vi "AlliGator Decay Fit Parameter Map Actions.vi"(0 "AlliGator Q Elements in":T4[](array[typedef]), 1 "VI in":refnum<vi>, 2 "Script in":bool, 5 "data value reference":refnum<data-value>, 7 "AlliGator Q Event in":T5=enum."GUI:Idle", 9 "Data":variant, 11 "error in (no error)":errorcluster, 12 "AlliGator Ctrl Refnums":T6) -> (3 "Script out":bool, 4 "AlliGator Q Elements out":T4[](array[typedef]), 6 "Data Value Reference out":refnum<data-value>, 10 "[Notebook Message]":T1[](array[typedef]) {"Message Style"."Text Alignment" items=["Left", "Right", "Center"]}, 15 "error out":errorcluster)   [LabVIEW 2021, in "AlliGator Action Engine.lvlib"]
doc: "Processes AlliGator decay fit parameter map-related actions."
uses:
  AlliGator Action Engine.lvlib
  AlliGator Internal Variables v2.ctl
  <vilib>/vision/Image Controls.llb/IMAQ Image.ctl
  AlliGator Gate Image Set.ctl
  AlliGator FLI Dataset Type.ctl
  AlliGator Data Series Type.ctl
  AlliGator Dataset Channel.ctl
  AlliGator Gate Arithmetic.ctl
  AlliGator Displayed Image.ctl
  Image/Named ROI Description.ctl
  AlliGator Decay Metadata v3.ctl
  AlliGator Decay Background Subtraction Info.ctl
  AlliGator Baseline Subtraction Method.ctl
  Graphs/XY Graph/XY Graph Plot Shift Parameters.ctl
  Graphs/XY Graph/XY Graph Plot Shift Method.ctl
  AlliGator Decay Extrapolation Parameters.ctl
  Phasor/Calibration Phasor (m, phi).ctl
  Phasor/Phasor Reference Series.ctl
  Phasor/Phasor Calibration Map v2.ctl
  Phasor/Phasor (g, s).ctl
  AlliGator Raw Phasor Plot Data v4.ctl
  Phasor/Phasor Standard Deviation Options.ctl
  AlliGator Phasor Multi-Harmonic Data.ctl
  Phasor/Phasor Harmonic Data.ctl
  AlliGator Decay Fit Options & Parameters v2.ctl
  Fits/IRF(X)PSED/Decay Fit Options v2.ctl
  Fits/Decay Convolution/Decay Model.ctl
  Fits/Residual Type.ctl
  Fits/IRF(X)PSED/Fit Weights Type.ctl
  Fits/Non-linear Fitting Method v2.ctl
  Fits/Fit Calculation Method.ctl
  Fits/Non-linear Fitting Algorithm.ctl
  AlliGator Decay Fit Parameter Constraints 2.ctl
  Fits/IRF(X)PSED/Decay Fit Parameters In List.ctl
  Fits/IRF(X)PSED/MLE Baseline Offset Type.ctl
  AlliGator Decay Preprocessing Parameters.ctl
  Fits/IRF(X)PSED/Decay Fit Parameters & Derived Quantities List.ctl
  AlliGator Q Event.ctl
  AlliGator Ctrl Refnums.ctl
  AlliGator Other Ctrl Refnums.ctl
  AlliGator State Indicator.ctl
  AlliGator Phasor Plot Ctrl Refnums.ctl
  AlliGator Phasor Graph Ctrl Refnums.ctl
  Phasor/Phasor Calibration Type.ctl
  AlliGator Dataset Ctrl Refnums.ctl
  AlliGator Registered Events Ctrl Refnums.ctl
  AlliGator Image Histogram Control Refnums.ctl
  Histograms/Linear Histogram Options.ctl
  Histograms/Histogram Bin Option.ctl
  Histograms/Histogram Bin Position.ctl
  AlliGator Decay Fit Map Control Refnums.ctl
  AlliGator Q Element.ctl
  Notebook/Notebook Message Object.ctl
  Rich Text Box/Text Formatting.ctl
  Rich Text Box/Text Colors.ctl
  Alligator Elements Order in Action Stack.ctl
  AlliGator Variables List.ctl
  AlliGator Image Display Type.ctl
  Palette/Image Palette Information.ctl
  Image/Image Display Palette Type.ctl
  Files/Load-Save File Info.ctl
  c5217346-0728-4db9-a30e-52dae72b7cfc.vi
  Variant/Variant to Data/Variant to Boolean.vi
  AlliGator Add Single Action to Stack.vi
  Variant/Variant to Data/Variant to [String].vi
  Variant/Variant to Data/Variant to String.vi
  Variant/Variant to Data/Variant to I32.vi
  AlliGator Local Decay Window.lvlib
  Fits/Fits.lvlib
  Rich Text Box/Rich Text Box.lvlib
  GUI/GUI.lvlib
  AlliGator Decay Fit Parameter Map.lvlib
  Variant/Variant to Data/Variant to Data.lvlib
  AlliGator Globals, Variables & Constants.lvlib
  Palette/Palette.lvlib
  AlliGator GUI.lvlib
  Image/Image.lvlib
  AlliGator Files.lvlib
  AlliGator Internal Variables.lvlib
  Files/Files.lvlib
  Sound/Sound.lvlib
  Phasor/Phasor.lvlib
  AlliGator Decay Preprocessing.lvlib
  Graphs/XY Graph/XY Graph Add-Ons.lvlib
  AlliGator Phasor Graph.lvlib
  AlliGator Phasor Plot.lvlib
  AlliGator Source Image.lvlib
  AlliGator Decay Fit.lvlib
  AlliGator Settings.lvlib
  AlliGator Dual-Channel Datasets.lvlib
  Histograms/Histogram Window.lvlib
  Notebook/Notebook.lvlib
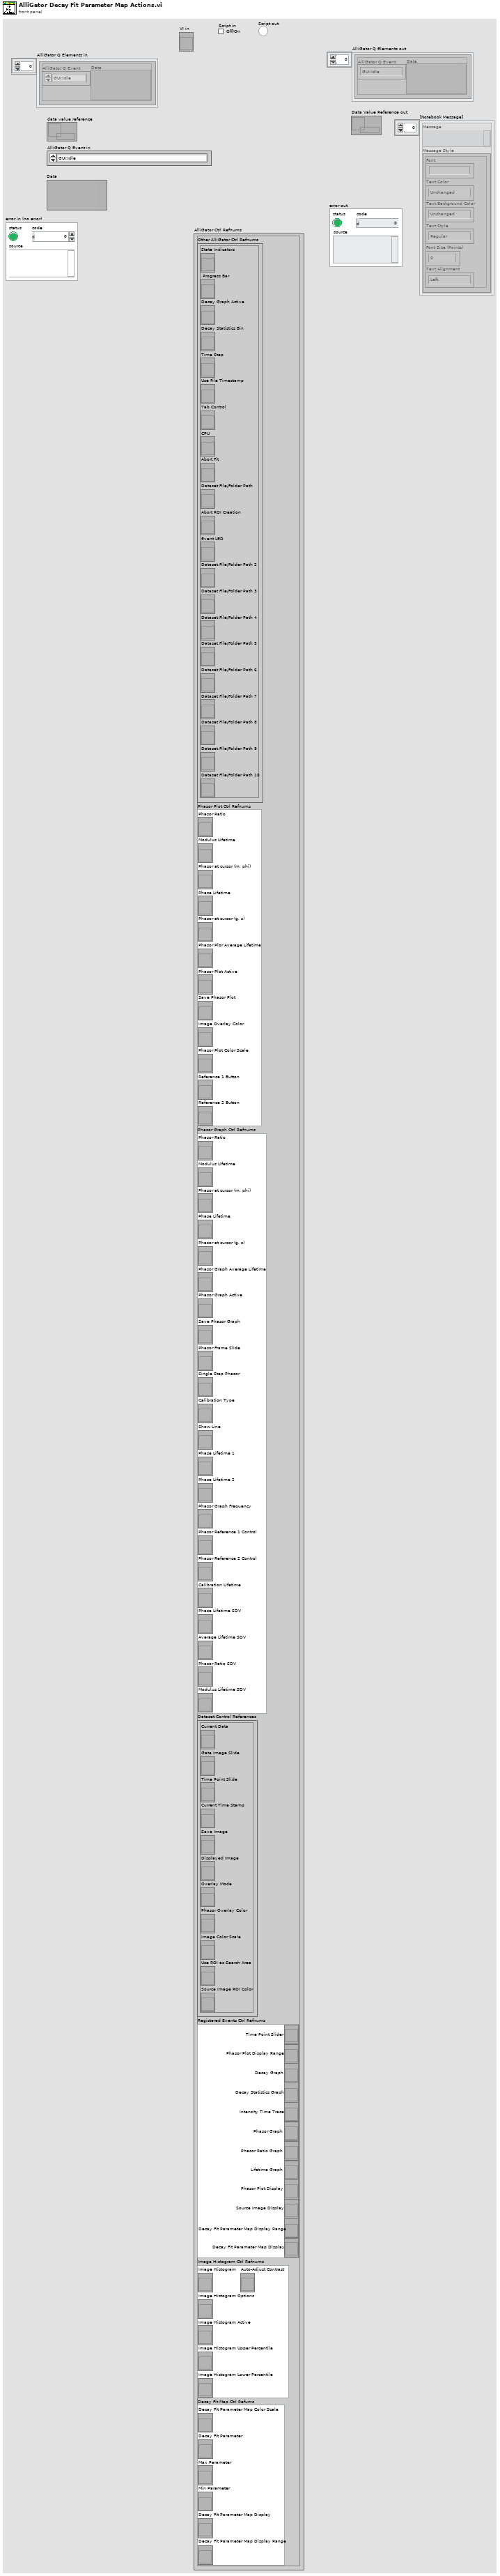
[diagram p1: front panel]
types:
  T1 = typedef "Notebook.lvlib/Notebook Message Object.ctl" = cluster{"Message":string, "Message Style":T2}
  T2 = typedef "Rich Text Box.lvlib/Text Formatting.ctl" = cluster{"Font":string, "Text Color":T3, "Text Background Color":T3, "Text Style":enum16{"Regular", "Bold", "Italic", "Underline", "Strikeout"}, "Font Size (Points)":dbl, "Text Alignment":i32}
  T3 = typedef "Rich Text Box.lvlib/Text Colors.ctl" = enum16{"Unchanged", "Black", "Blue", "Brown", "Gray", "Green", "Orange", "Pink", "Red", "White"}
  T4 = typedef "AlliGator Action Engine.lvlib/AlliGator Q Element.ctl" = cluster{"AlliGator Q Event":T5, "Data":variant}
  T5 = typedef "AlliGator Action Engine.lvlib/AlliGator Q Event.ctl" = enum16{"---- Files ----", "Files:Set Batch Export Files To Save", "Files:Set Dataset Loading & Pre-processing Options", "Files:Check #Frames in Dataset", "Files:Increment Frame Index", "Files:Open Mask Image", "Files:Open White Light Image", "Files:Open Single Dataset", "Files:New Folder of Folders Selected", "Files:Load File (all Types)_Scriptable", "Files:Move Flattened Series to Folders Series", "Files:Select Folder", "Files:Load FLI Dataset", "Files:Load Swiss SPAD 1 Dataset", "Files:Load Swiss SPAD 2 Dataset", "Files:Load .sdt FLI Dataset", "Files:Load .ptu FLI Dataset", "Files:Load .bin FLI Dataset", "Files:Load Single Gate Image Folder", "Files:Load I/m/phi Dataset (deprecated)", "Files:Load Single Image", "Files:Subtract Background File", "Files:Export FLI Dataset", "Files:Load HDF5 FLI Dataset", "Files:Set Destination File Path", "Files:Save Mask Image", "Files:Batch Conversion", "Files:New Folder Selected", "Files:Close FLI Dataset", "Files:Close FLI Dataset Series", "Files:Close White Light Image", "Files:Close Mask Image", "---- FLI Dataset ----", "FLI Dataset:Channel Arithmetic", "FLI Dataset:Export Average Lifetime Map as ASCII", "FLI Dataset:Export User-Defined Quantity Map as ASCII", "FLI Dataset:Python Function FLI Dataset Event", "FLI Dataset:ROI Analysis", "FLI Dataset:Tilted Logistic Square Gated IRF Characteristics Map", "FLI Dataset:Logistic Square Gated IRF Characteristics Map", "FLI Dataset:Square Gated IRF Characteristics Map", "FLI Dataset:Multi-ROI Single-Pixel Phasor Analysis", "FLI Dataset:Multi-ROI Single-Pixel NLSF Analysis", "FLI Dataset:All ROIs IRF Extraction", "FLI Dataset:All ROIs Decay Fit Non-Interactive (Fast + Individual IRF)", "FLI Dataset:All ROIs Phasor Analysis", "FLI Dataset:All ROIs Decay Fit", "FLI Dataset:Fluorescence Decay Statistics", "FLI Dataset:Update Decay Statistics Graph", "FLI Dataset:Get Decay from ROI", "FLI Dataset:All ROIs Average Lifetimes", "---- FLI Dataset Series ----", "FLI Dataset Series:Sum All Datasets in Series", "FLI Dataset Series:Add Dataset to Accumulated Dataset", "FLI Dataset Series:Display Accumulated Dataset", "FLI Dataset Series:Clear Dataset Series Sum", "FLI Dataset Series:Time-Series Analysis (NLSF)", "FLI Dataset Series:Time-Series Analysis (Phasor)", "---- Image ----", "Image:Update Image Profile Plots", "Image:Image Histogram Cursor Move", "Image:Image Histogram", "Image:Image Contrast", "Image:Set Image Histogram Cursor Move Flag", "Image:Clear Image Overlay", "Image:Use ROI as Search Area", "Image:Set ROI Diameter", "Image:Save Image Data as TIFF", "Image:Save Displayed Image with Overlay", "Image:Save Image Overlay Only", "Image:Save Image as Hot Pixel Mask", "Image:Change Source Image Color Palette", "Image:Copy Image to Clipboard", "Image:Source Image ROI Selection", "Image:Delete All ROIs", "Image:Delete All Unselected ROIs", "Image:Delete ROI", "Image:Merge All ROIs", "Image:Store ROI", "Image:Source Image ROI Storage", "Image:Export ROI Description to Notebook", "Image:Save ROI", "Image:Load ROI", "Image:Paste ROI Definition", "Image:Clear ROI", "Image:Identify ROIs in Mask Image", "Image:Create Complementary ROI", "Image:Create Contour ROI", "Image:Create ROI(s) from Pixels with Peak above Min_Scriptable", "Image:Create ROI(s) from Pixels with Intensity above Min_Scriptable", "Image:Compute ROI Statistics", "Image:Delete ROI(s) based on ROI Characteristics", "Image:Create ROI Grid", "Image:ROI to Individual Pixel ROIs", "Image:Python Function Source Image Event", "Image:Show Phasor Calibration Map ROI Centers", "Image:Convert ROI to Mask Image", "Image:Mouse Move", "Image:Mouse Up", "Image:Set Source Image Mouse Move Flag", "Image:Add Scale Bar Overlay", "Image:Delete Existing ROIs Option", "---- Decay ----", "Decay:Clear IRF/Reference Plot", "Decay:Clear Local IRFs", "Decay:Add Decay to Graph", "Decay:Smoothen Plot", "Decay:Smoothen Plot Tail", "Decay:Average Selected Plots", "Decay:Extract IRF", "Decay:Optimal IRF Extraction", "Decay:Threshold IRF", "Decay:Fit to Model IRF", "Decay:Fit IRF to Square Gate", "Decay:Fit IRF to Logistic Square Gate", "Decay:Fit IRF to Tilted Logistic Square Gate", "Decay:Create Bounding Cursors Set", "Decay:Export Bounding Cursors Definition to Notebook", "Decay:Denoise Plot", "Decay:Compute Cumulative Function", "Decay:Use as Reference Decay", "Decay:Show Reference Decay/IRF", "Decay:Extrapolate Decay", "Decay:Create Head & Tail Bounding Cursors", "Decay:Store Cursor-defined Head & Tail Fractions", "Decay:Rebin Plot", "Decay:1-Normalize Decay", "Decay:[0-1]-Normalize Plot", "Decay:Straighten Decay", "Decay:Shift Decay", "Decay:Fold Decay", "Decay:Fit Decay", "Decay:Global Fit of Selected Decays", "Decay:Post Global Fit Script", "Decay:Add Global Fit Parameters to Graph", "Decay:Add Decay Parameter(s) to Plot (Graph)", "Decay:Export Decay to Phasor Graph", "Decay:Plot Decay Shifts", "Decay:Compute Average Lifetime", "Decay:Plot Convolution", "Decay:Graph Tip Strip Update", "---- Decay Statistics ----", "Decay Statistics:Tip Strip Update", "---- Intensity Time Trace ----", "Intensity Time Trace:Use File Timestamp", "Intensity Time Trace:Load Intensity Corrections File", "Intensity Time Trace:Clear Intensity Corrections File", "Intensity Time Trace:Tip Strip Update", "---- Phasor Plot ----", "Phasor Plot:Build Phasor Plot", "Phasor Plot:Change Phasor Plot Color Palette", "Phasor Plot:Adjust Phasor Plot Display Range", "Phasor Plot:Highlight Image ROI in Phasor Plot", "Phasor Plot:Save Phasor Plot Image with Overlay", "Phasor Plot:Export Complex Phasor Map", "Phasor Plot:Export Phasor Ratio Map", "Phasor Plot:Export Average Lifetime Map", "Phasor Plot:Compute Phase Lifetime Histogram", "Phasor Plot:Compute Phasor Ratio Histogram", "Phasor Plot:Compute Phase Lifetime vs Intensity Scatter Plot", "Phasor Plot:Weber 2-Component Decomposition", "Phasor Plot:Update Phasor Color Map Vertices", "Phasor Plot:Clear Phasor Overlay", "Phasor Plot:Use Segment Extremities as References", "Phasor Plot:Use UC/Segment Intersections as References", "Phasor Plot:Use UC/Principal Axis Intersections as References", "Phasor Plot:Use UC/Linear Fit Intersections as References", "Phasor Plot:Update Phasor Plot Reference", "Phasor Plot:Show Local Phasor Info in Phasor Plot", "Phasor Plot:Update Phasor Plot State", "Phasor Plot:Phasor Plot ROI Storage", "Phasor Plot:Phasor Plot ROI Selection", "Phasor Plot:Python Function Phasor Plot Event", "Phasor Plot:Overlay Phasor ROI, Ratio or Map in Source Image", "Phasor Plot:Compute Decay of Selected Phasors", "Phasor Plot:Phasor at Image Pixel", "Phasor Plot:Mouse Move", "Phasor Plot:Mouse Up", "Phasor Plot:Display Range Mouse Move", "Phasor Plot:Set Mouse Move Flag", "---- Phasor Graph ----", "Phasor Graph:Calibrated Phasor Map Series", "Phasor Graph:Whole Image Phasor Scatter Plot (Todo)", "Phasor Graph:Get Phasor Value", "Phasor Graph:Create New Phasor Plot Dialog", "Phasor Graph:Update Last Phasor Value", "Phasor Graph:Update Phasor (m, phi)", "Phasor Graph:Remove Single Phasor from Plot", "Phasor Graph:Add Single Phasor to Plot", "Phasor Graph:Remove Phasor Plot", "Phasor Graph:Remove Selected Phasor Plots", "Phasor Graph:Clear Phasor Data", "Phasor Graph:Clear Phasor Graph", "Phasor Graph:Cursor Move", "Phasor Graph:Draw Cursor Connecting Line", "Phasor Graph:Clear Cursor Connecting Line", "Phasor Graph:Find UC Intersection", "Phasor Graph:Use UC/Cursor-Defined Line Intersections", "Phasor Graph:Use Selected Plots Fitted Line/UC Intersections", "Phasor Graph:Use Selected Plots Principal Axis/UC Intersections", "Phasor Graph:Show Single Phasor", "Phasor Graph:Save Single Phasor Plot", "Phasor Graph:Save All Phasor Plots", "Phasor Graph:Load Phasor Plot(s)", "Phasor Graph:Phasor Multiplication", "Phasor Graph:Compute Average Phasor", "Phasor Graph:Compute Multiple Average Phasors (Selected Plots)", "Phasor Graph:Export Single Phasor Plot Phase Lifetimes", "Phasor Graph:Phase Lifetime Trajectory", "Phasor Graph:Phase Lifetime vs Intensity Scatter Plot (deprecated)", "Phasor Graph:Parameter 2 vs Parameter 1 Scatter Plot", "Phasor Graph:Use Cursor n Location", "Phasor Graph:Set Reference n to Current Phase Lifetime Value", "Phasor Graph:Set Reference n to Lifetime Value", "Phasor Graph:Set Cursor n Location", "Phasor Graph:Save Phasor Graph Image", "Phasor Graph:Update SEPL Plot", "Phasor Graph:Export Single Phasor Plot Data", "Phasor Graph:Export Selected Phasor Plots Data", "Phasor Graph:Python Function Phasor Graph Event", "Phasor Graph:Tip Strip Update", "---- Calibration ----", "Calibration:Set Calibration Type", "Calibration:Load/Save Phasor Calibration", "Calibration:Load/Save Phasor Calibration Series", "Calibration:Load/Save Phasor Calibration Map", "Calibration:Use as Calibration", "Calibration:Compute Optimal Calibration from Phasor References", "Calibration:Clear Phasor Calibration", "Calibration:Single Phasor Calibration Information", "Calibration:Use as Calibration Series", "Calibration:Use as Calibration Map", "Calibration:Clear Calibration Series", "Calibration:Phasor Calibration Series Information", "Calibration:Clear Calibration Map", "Calibration:Phasor Calibration Map Information", "Calibration:Apply Phasor Calibration", "Calibration:Update Single Plot Calibration", "Calibration:Update Multiple Plots Calibration", "Calibration:Clear Single Plot Calibration", "Calibration:Clear All Plots Calibrations", "Calibration:Clear Plot(s) Calibration(s)?", "Calibration:Phasor Calibration Maps (# Gates Series)", "---- Phasor Ratio ----", "Phasor Ratio:Clear Reference n", "Phasor Ratio:Toggle Selected Plot(s)  Lock to Reference 1", "Phasor Ratio:Use as Reference n", "Phasor Ratio:Send Reference n to Notebook", "Phasor Ratio:Toggle Selected Plot(s)  Lock to Reference 2", "Phasor Ratio:Compute Phasor Ratio at Mouse Location", "Phasor Ratio:Compute Phasor Plot's Average Phasor Ratio", "Phasor Ratio:Compute Time-Series Phasor Ratios", "Phasor Ratio:Fit Line to Phasor Ratio Plot", "Phasor Ratio:Save References", "Phasor Ratio:Load References", "Phasor Ratio:Update Phasor Reference 1", "Phasor Ratio:Update Phasor Reference 2", "Phasor Ratio:Move Cursor n to Reference n", "Phasor Ratio:Use as Phasor Reference 1 Lifetime", "Phasor Ratio:Use as Phasor Reference 2 Lifetime", "Phasor Ratio:Export Phasor Ratio Map as ASCII", "Phasor Ratio:Tip Strip Update", "---- Lifetime & Other Parameters Graph ----", "Lifetime:Tip Strip Update", "---- Decay Fit Parameter Map ----", "Decay Fit Parameter Map:Export ROI NLSF Data as ASCII", "Decay Fit Parameter Map:Set Decay Fit  Parameter Map Selection", "Decay Fit Parameter Map:Build Decay Fit Parameter Map", "Decay Fit Parameter Map:Change Decay Fit Parameter Map Color Palette", "Decay Fit Parameter Map:Export Decay Fit Parameter Map Data as ASCII", "Decay Fit Parameter Map:Export All Decay Fit Parameter Maps Data as ASCII", "Decay Fit Parameter Map:Send Map Data to Lifetime Graph", "Decay Fit Parameter Map:Save Decay Fit Parameter Map Image", "Decay Fit Parameter Map:Save-Load IRFs & Fit Data", "Decay Fit Parameter Map:Update Local Decay Plots", "Decay Fit Parameter Map:Python Function Decay Fit Parameters Map Event", "Decay Fit Parameter Map:Overlay Decay Fit Parameter Map in Source Image", "Decay Fit Parameter Map:Plot Map Data vs Intensity", "Decay Fit Parameter Map:Mouse Up", "Decay Fit Parameter Map:Display Range Mouse Move", "---- Generic Graph ----", "Generic Graph:Generic XY Graph Event", "Generic Graph:Python Function XY Graph Event", "Generic Graph:New Plot", "Generic Graph:Save Plot", "Generic Graph:XY Plot Histogram", "Generic Graph:Set XY Graph Plot Name", "Generic Graph:Set Last Cursor Style", "Generic Graph:Tip Strip Update", "---- GUI ----", "GUI:Start Script", "GUI:Type of Displayed Image Changed", "GUI:Gate Image Slide Changed", "GUI:Show Busy Icon", "GUI:Show Busy Icon & Abort Button", "GUI:Hide Busy Icon", "GUI:Hide Busy Icon & Abort Button", "GUI:Abort", "GUI:End Script", "GUI:Start Timing", "GUI:End Timing", "GUI:Set State Indicator", "GUI:Send Parameters JSON Strings to Clipboard", "GUI:Set Gate Step", "GUI:Idle", "GUI:Initialization", "GUI:Quit", "GUI:Increment Dataset Index", "GUI:Set Dataset Index to -1", "GUI:Time Series Slider Moved", "GUI:Time Series Slider Changed", "GUI:Toggle Playback or Loop", "GUI:Playback Script", "GUI:Set Phasor Frequency", "GUI:Open Window", "GUI:Start Test Script", "GUI:End Test Script", "DEBUG"}
  T6 = typedef "AlliGator GUI.lvlib/AlliGator Ctrl Refnums.ctl" = cluster{"Other AlliGator Ctrl Refnums":T7, "Phasor Plot Ctrl Refnums":T8, "Phasor Graph Ctrl Refnums":T9, "Dataset Control References":T10, "Registered Events Ctrl Refnums":T11, "Image Histogram Ctrl Refnums":T12, "Decay Fit Map Ctrl Refums":T13}
  T7 = typedef "AlliGator GUI.lvlib/AlliGator Other Ctrl Refnums.ctl" = cluster{"State Indicators":refnum<vi>, " Progress Bar":refnum<vi>, "Decay Graph Active":refnum<vi>, "Decay Statistics Bin":refnum<vi>, "Time Step":refnum<vi>, "Use File Timestamp":refnum<vi>, "Tab Control":refnum<vi>, "CPU":refnum<vi>, "Abort Fit":refnum<vi>, "Dataset File/Folder Path":refnum<vi>, "Abort ROI Creation":refnum<vi>, "Event LED":refnum<vi>, "Dataset File/Folder Path 2":refnum<vi>, "Dataset File/Folder Path 3":refnum<vi>, "Dataset File/Folder Path 4":refnum<vi>, "Dataset File/Folder Path 5":refnum<vi>, "Dataset File/Folder Path 6":refnum<vi>, "Dataset File/Folder Path 7":refnum<vi>, "Dataset File/Folder Path 8":refnum<vi>, "Dataset File/Folder Path 9":refnum<vi>, "Dataset File/Folder Path 10":refnum<vi>}
  T8 = typedef "AlliGator GUI.lvlib/AlliGator Phasor Plot Ctrl Refnums.ctl" = cluster{"Phasor Ratio":refnum<vi>, "Modulus Lifetime":refnum<vi>, "Phasor at cursor (m, phi)":refnum<vi>, "Phase Lifetime":refnum<vi>, "Phasor at cursor (g, s)":refnum<vi>, "Phasor Plor Average Lifetime":refnum<vi>, "Phasor Plot Active":refnum<vi>, "Save Phasor Plot":refnum<vi>, "Image Overlay Color":refnum<vi>, "Phasor Plot Color Scale":refnum<vi>, "Reference 1 Button":refnum<vi>, "Reference 2 Button":refnum<vi>}
  T9 = typedef "AlliGator GUI.lvlib/AlliGator Phasor Graph Ctrl Refnums.ctl" = cluster{"Phasor Ratio":refnum<vi>, "Modulus Lifetime":refnum<vi>, "Phasor at cursor (m, phi)":refnum<vi>, "Phase Lifetime":refnum<vi>, "Phasor at cursor (g, s)":refnum<vi>, "Phasor Graph Average Lifetime":refnum<vi>, "Phasor Graph Active":refnum<vi>, "Save Phasor Graph":refnum<vi>, "Phasor Frame Slide":refnum<vi>, "Single Step Phasor":refnum<vi>, "Calibration Type":refnum<vi>, "Show Line":refnum<vi>, "Phase Lifetime 1":refnum<vi>, "Phase Lifetime 2":refnum<vi>, "Phasor Graph Frequency":refnum<vi>, "Phasor Reference 1 Control":refnum<vi>, "Phasor Reference 2 Control":refnum<vi>, "Calibration Lifetime":refnum<vi>, "Phase Lifetime SDV":refnum<vi>, "Average Lifetime SDV":refnum<vi>, "Phasor Ratio SDV":refnum<vi>, "Modulus Lifetime SDV":refnum<vi>}
  T10 = typedef "AlliGator GUI.lvlib/AlliGator Dataset Ctrl Refnums.ctl" = cluster{"Current Data":refnum<vi>, "Gate Image Slide":refnum<vi>, "Time Point Slide":refnum<vi>, "Current Time Stamp":refnum<vi>, "Save Image":refnum<vi>, "Displayed Image":refnum<vi>, "Overlay Mode":refnum<vi>, "Phasor Overlay Color":refnum<vi>, "Image Color Scale":refnum<vi>, "Use ROI as Search Area":refnum<vi>, "Source Image ROI Color":refnum<vi>}
  T11 = typedef "AlliGator GUI.lvlib/AlliGator Registered Events Ctrl Refnums.ctl" = cluster{"Time Point Slider":refnum<vi>, "Phasor Plot Display Range":refnum<vi>, "Decay Graph":refnum<vi>, "Decay Statistics Graph":refnum<vi>, "Intensity Time Trace":refnum<vi>, "Phasor Graph":refnum<vi>, "Phasor Ratio Graph":refnum<vi>, "Lifetime Graph":refnum<vi>, "Phasor Plot Display":refnum<vi>, "Source Image Display":refnum<vi>, "Decay Fit Parameter Map Display Range":refnum<vi>, "Decay Fit Parameter Map Display":refnum<vi>}
  T12 = typedef "AlliGator GUI.lvlib/AlliGator Image Histogram Control Refnums.ctl" = cluster{"Image Histogram":refnum<vi>, "Image Histogram Options":refnum<vi>, "Image Histogram Active":refnum<vi>, "Image Histogram Upper Percentile":refnum<vi>, "Image Histogram Lower Percentile":refnum<vi>, "Auto-Adjust Contrast":refnum<vi>}
  T13 = typedef "AlliGator Decay Fit Parameter Map.lvlib/AlliGator Decay Fit Map Control Refnums.ctl" = cluster{"Decay Fit Parameter Map Color Scale":refnum<vi>, "Decay Fit Parameter":refnum<vi>, "Max Parameter":refnum<vi>, "Min Parameter":refnum<vi>, "Decay Fit Parameter Map Display":refnum<vi>, "Decay Fit Parameter Map Display Range":refnum<vi>}
  T14 = typedef "AlliGator Action Engine.lvlib/Alligator Elements Order in Action Stack.ctl" = enum16{"Enqueue 2 AFTER 1", "Enqueue 2 BEFORE 1"}
  T15 = typedef "Image.lvlib/AlliGator Image Display Type.ctl" = enum16{"Source Image", "Phasor Plot", "Decay Fit Parameter Map"}
  T16 = typedef "AlliGator Globals, Variables & Constants.lvlib/AlliGator Variables List.ctl" = enum16{"---- GUI ----", "Initialization Status", "State Indicators Refnum", "Original AlliGator Menu Items", "Current Action Loop State", "Script in progress", "Playback", "Loop Playback", "Search ROI Used", "Search ROI", "Decay Graph Max Legend Size", "Intensity Graph Max Legend Size", "Decay Statistics Graph Max Legend Size", "Phasor Graph Max Legend Size", "Phasor Ratio Graph Max Legend Size", "Lifetime Graph Max Legend Size", "---- Files ----", "Export Dataset Frames as Individual Files", "Show Batch Export Help Balloons", "Frames in Dataset", "ptu File Frame Start Indices", "Current Frame in Dataset", "Current Frame Timestamp", "------ Python Plugins ------", "Python Plugins Information", "Python Session", "Valid Python Session?", "---- Source Image ----", "Dataset Loaded", "Dataset Metadata", "Dataset Channel", "Dataset Data Description", "Background Dataset Metadata", "Background Dataset Channel", "Background Dataset Data Description", "Background File Subtraction", "Background File Path", "Background File Pile-up Correction", "Background File Pixel Well Capacity", "Background File Scaling Factor", "Source Image ROIs", "Current Source Image ROI", "Source Image ROI Event Refnum", "X_Source Image Display Range", "X_Source Image Palette Information", "Source Image Palette List", "Source Image Scale", "Current Dataset Load Settings", "Source Image:ROI Overlay Color", "---- Image Profile Window ----", "Image Profile:Overlay ROI in Source Image", "Image Profile Window Event Refnum", "Image Profile:IntensityType", "Image Profile:Intensity Average Type", "Image Profile:Intensity-weighted SDV", "Image Profile:Box Profile Type", "Image Profile Window Open", "Image Profile:Plotted Fit Parameter", "X_Type of Displayed Image", "X_Time Gate Slider", "Dataset Path", "Source Image Overlay to Erase", "Is Displayed Image Accumulated", "White Light Image Modified", "Mask Image Modified", "Macrotime Gate Separation", "------ Phasor Graph -------", "Phasor Graph:Show Line", "---- Phasor Plot ---", "Phasor Plot Parameters Changed", "FLI Dataset Modified since last Phasor Plot Calculation", "Phasor Harmonics Data", "Selected Phasor Harmonics", "Phasor Harmonic Manager Event Refnum", "Phasor Plot ROIs", "Current Phasor Plot ROI", "Phasor Plot ROI Event Refnum", "Phasor Plot Image Reference Points", "Phasor Plot Computed", "Phasor Plot Palette Information", "Phasor Plot Palette List", "Phasor Ratio Palette Information", "Phasor Ratio Palette List", "Phasor Image Scale", "Phasor Plot Image Overlay to Erase", "Phasor Plot Image Elements to Update", "Current Phasor Plot Calculation Parameters", "Current Phasor Calibration Options", "Reset Cumulated Phasor Plot", "Phasor Ratio Reference 1", "Phasor Ratio Lifetime Reference 1", "Phasor Ratio Reference 1 Frequency", "Phasor Ratio Reference 2", "Phasor Ratio Lifetime Reference 2", "Phasor Ratio Reference 2 Frequency", "---- Decay Analysis ----", "Number of Selected Decays to Fit", "LS Fit Results", "LAR Fit Results", "BS Fit Results", "Last Decay Max - Min", "Best Fit Parameters", "Best Fit Parameter Names", "Actual Size X", "Actual Size Y", "Binning X", "Binning Y", "Actual # Gates", "Dataset Number", "Gates to...", "Gates Skipped", "Gates to keep", "Gate Step", "Gate Separation", "Reversed Gates", "Pile-up Correction", "Pixel Well Capacity", "Background Subtracted", "Background Subtraction Method", "Background Definition Range", "Background File (deprecated)", "Number of Dataset Accumulated", "Array of Accumulated Dataset Paths", "Do Averaged Datasets", "Destination File Path", "Process Plot Target", "Use 1/D as Phasor Frequency", "---- Decay Fit Parameter Map -----", "Decay Fit Parameter Map Palette Information", "Decay Fit Parameter Map Palette List", "Local Decay Graph Window Event Refnum", "------- Local Decay Window ---------", "Use normalized IRF for convolution", "----- Miscellaneous ----", "Skippable Dialog Windows Status"}
  T17 = typedef "Palette.lvlib/Image Palette Information.ctl" = cluster{"Palette Name [# Colors,int?,inv?]":string, "Palette Type":T18, "Palette Colors":u32[], "Interpolate?":bool}
  T18 = typedef "Image.lvlib/Image Display Palette Type.ctl" = u32
  T19 = typedef "Files.lvlib/Load-Save File Info.ctl" = cluster{"Load/Save":bool, "File Path":path}
  T20 = typedef "Fits.lvlib/Decay Fit Parameters & Derived Quantities List.ctl" = enum16{"Offset", "Baseline", "A_1", "tau_1", "A_2", "tau_2", "<tau>_a", "f1_a", "f2_a", "<tau>_i", "f1_i", "f2_i", "-", "R^2", "Chi^2"}
  T21 = typedef "AlliGator Decay Fit Parameter Map.lvlib/AlliGator Decay Parameter Map Update Event Data.ctl" = cluster{"Parameter":T20, "Parameter changed":bool}
  T22 = typedef "Image.lvlib/Image Save File Format.ctl" = enum16{"PNG", "JPEG", "BMP"}
  T23 = typedef "ROI Descriptor" = cluster{"Global Rectangle":i32[], "Contours":cluster{"ID":enum32{"External", "Internal"}, "Type":u32, "Coordinates":i32[]}[]}
  T24 = typedef "Image.lvlib/Image Control Refnum.ctl" = refnum<vi>
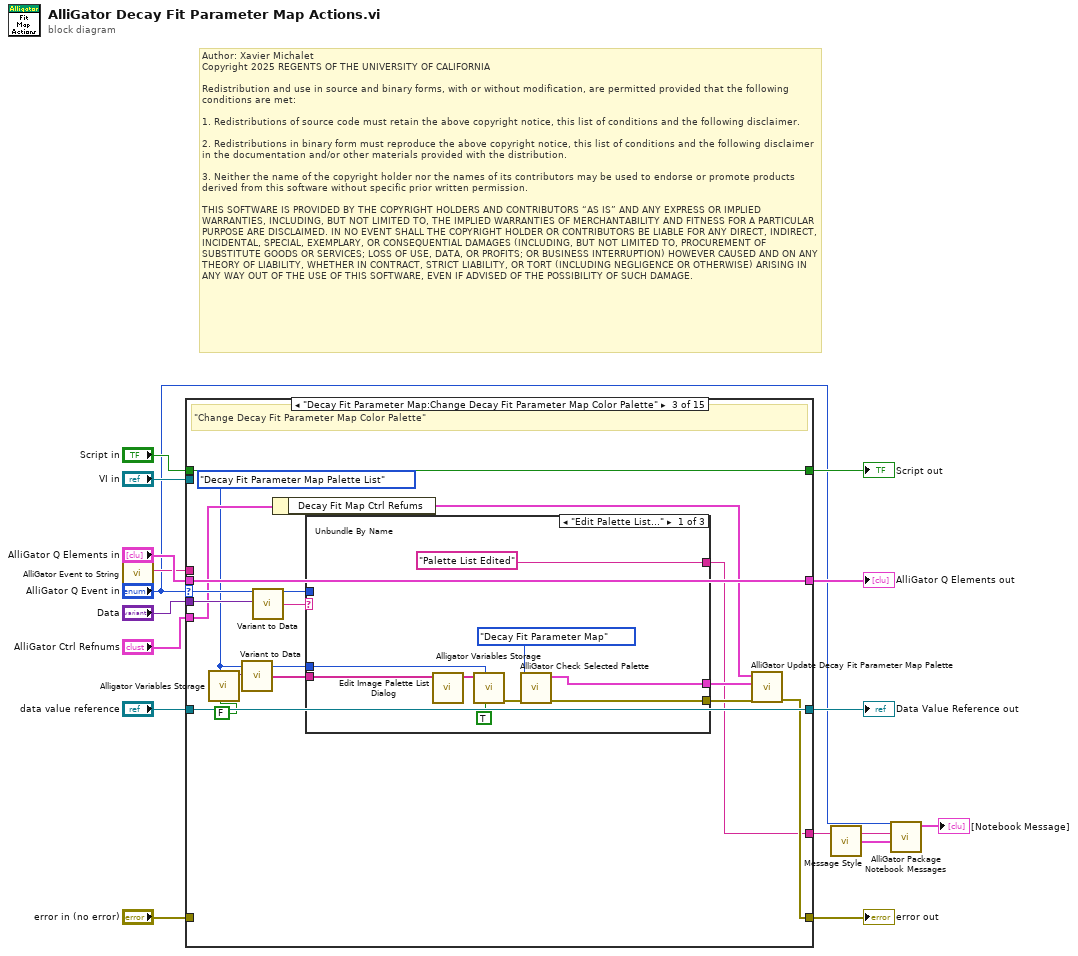
[diagram p0: block diagram]
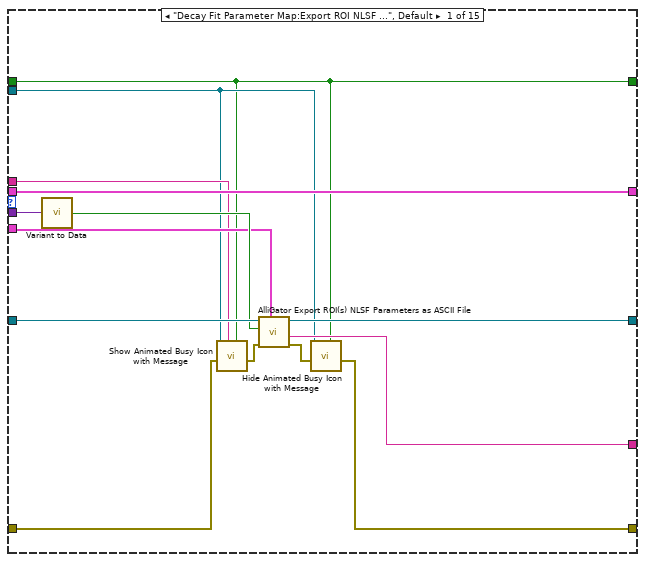
[diagram p2: hidden frame]
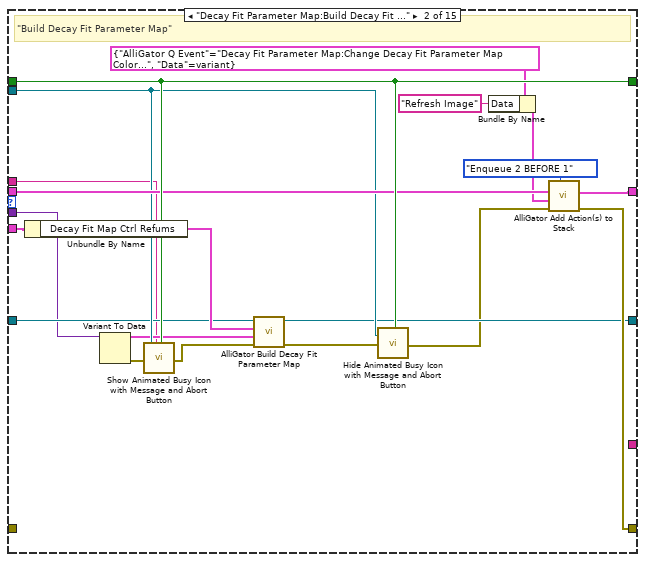
[diagram p3: hidden frame]
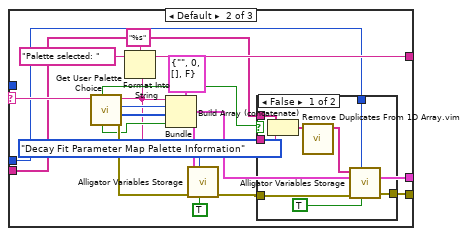
[diagram p4: hidden frame]
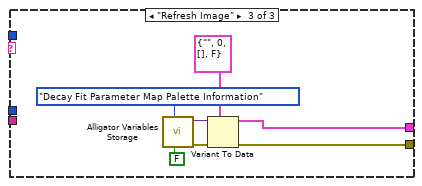
[diagram p6: hidden frame]
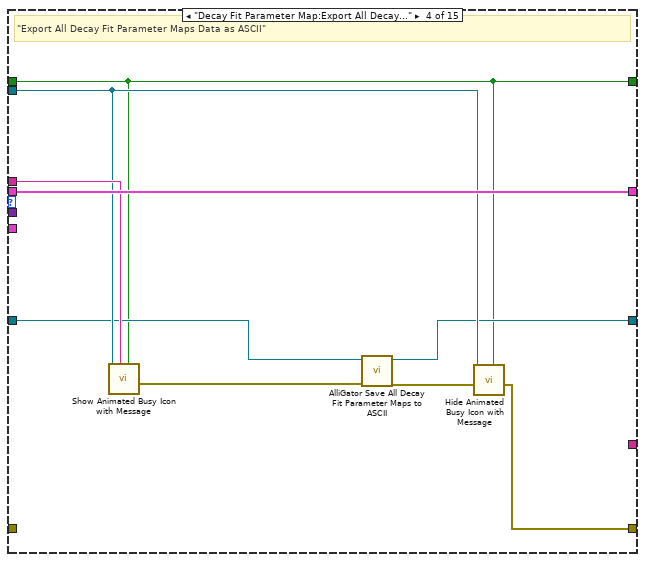
[diagram p7: hidden frame]
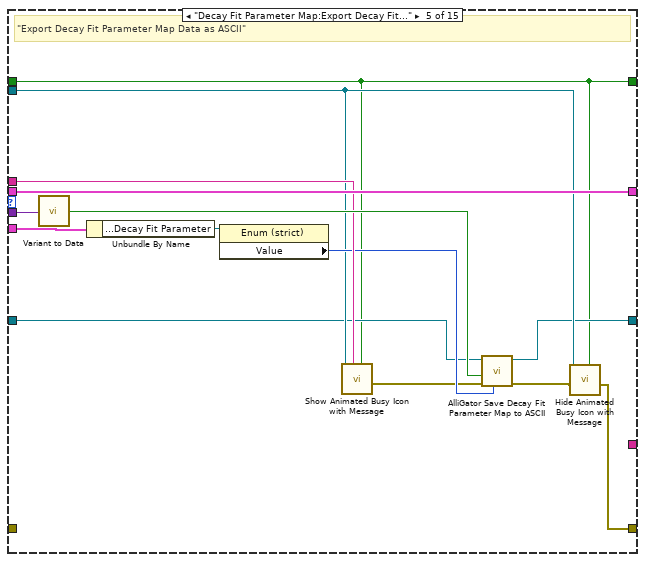
[diagram p8: hidden frame]
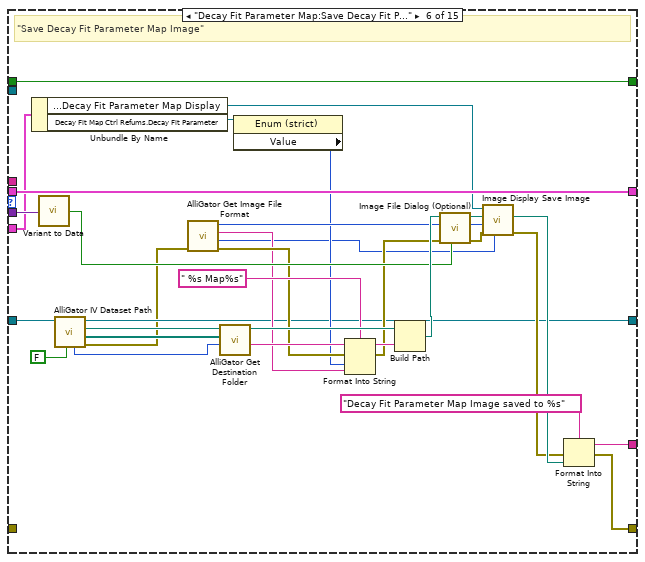
[diagram p9: hidden frame]
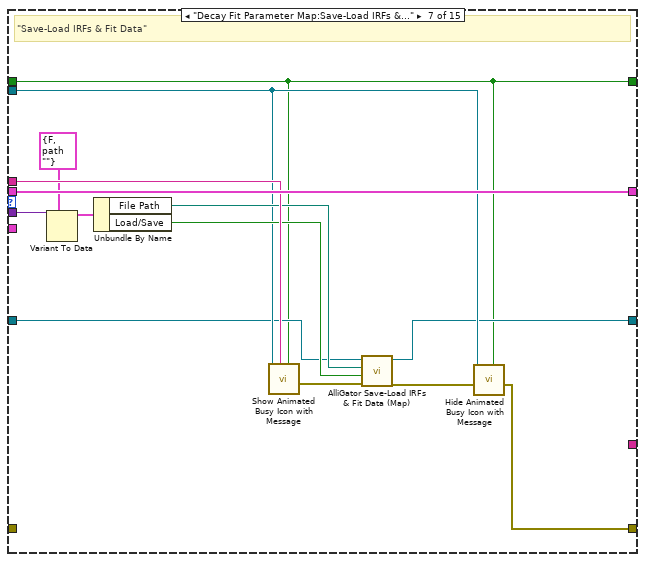
[diagram p10: hidden frame]
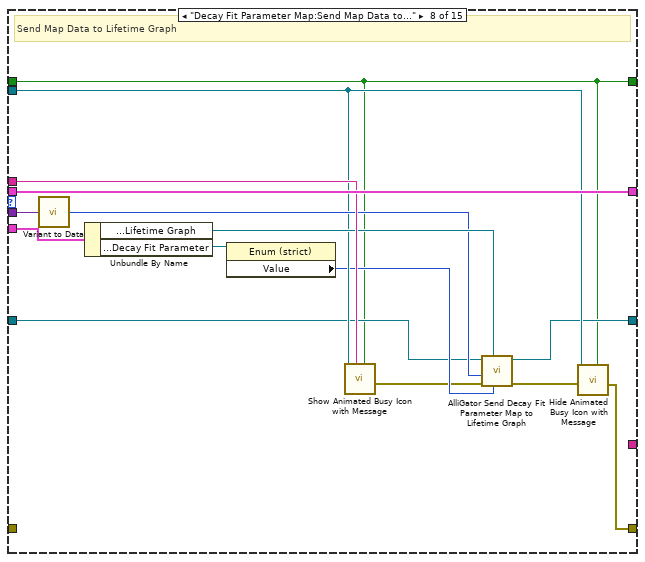
[diagram p11: hidden frame]
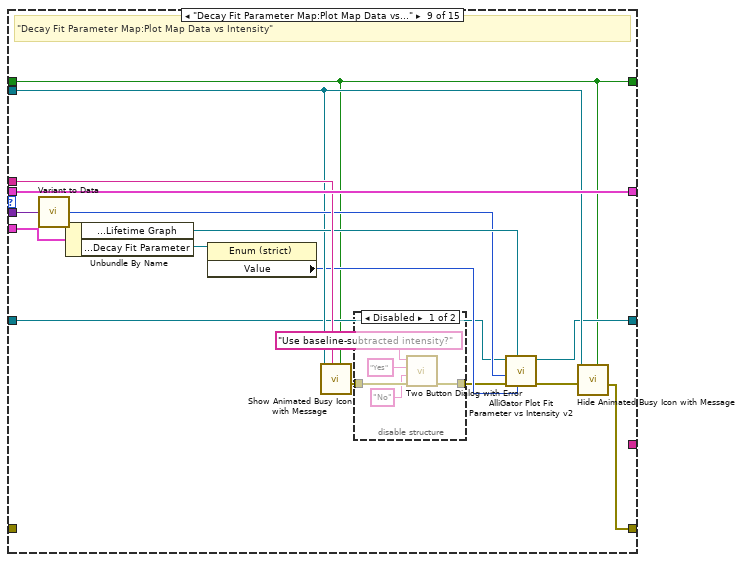
[diagram p12: hidden frame]
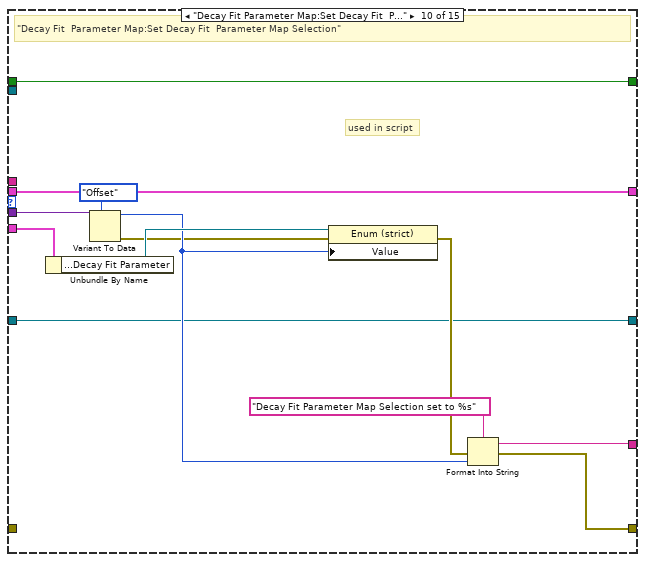
[diagram p14: hidden frame]
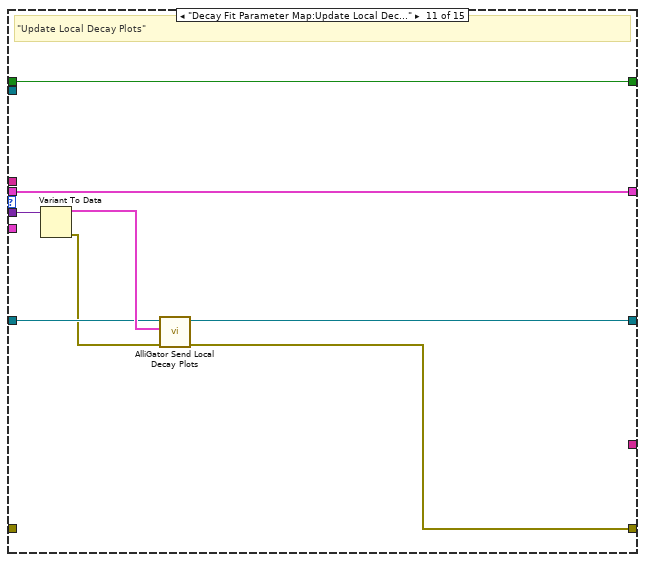
[diagram p15: hidden frame]
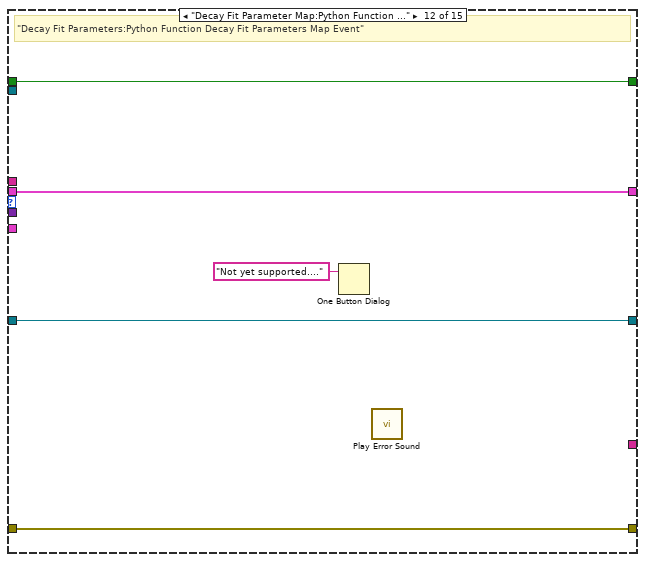
[diagram p16: hidden frame]
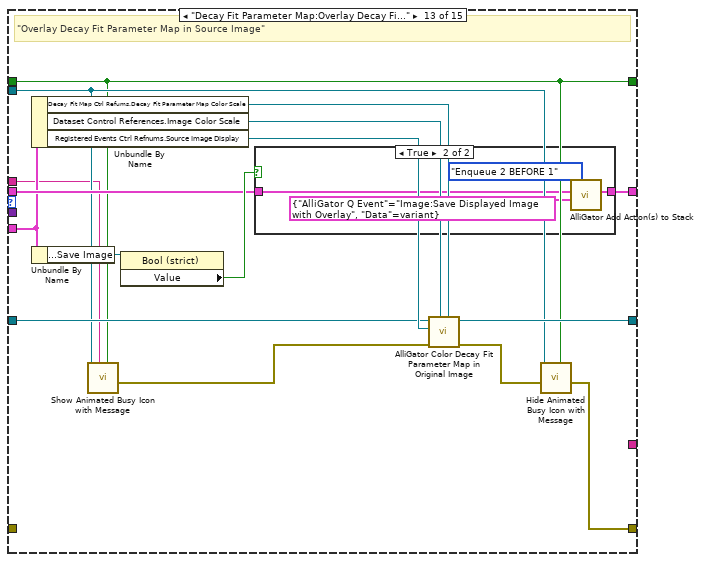
[diagram p17: hidden frame]
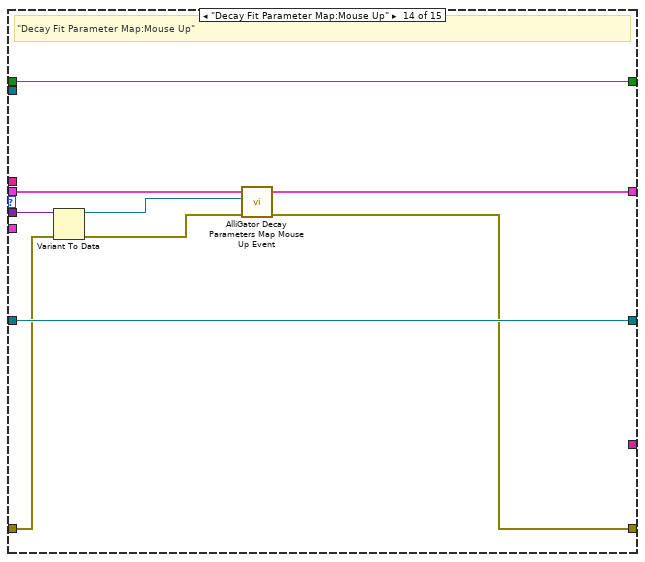
[diagram p19: hidden frame]
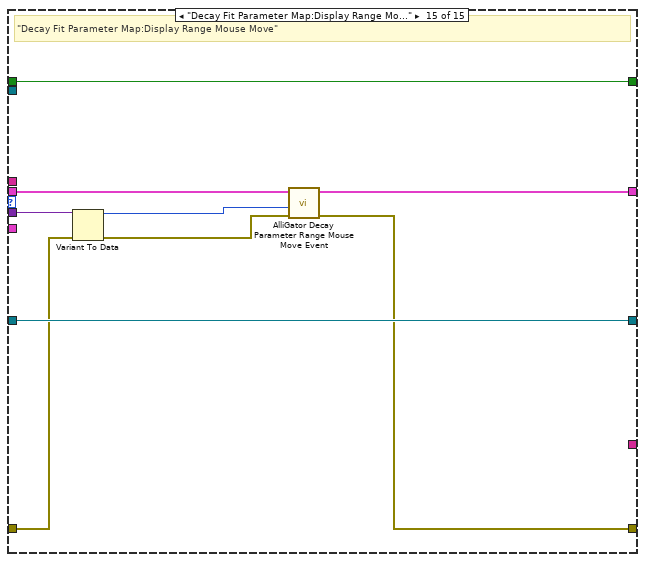
[diagram p20: hidden frame]
diagram:
  # "Author: Xavier Michalet\nCopyright 2025 REGENTS OF THE UNIVERSITY OF CALIFORNIA\n\nRedistribution and use in source and binary forms, with or without modification, are permitted provided that the following conditions are met:\n\n1. Redistributions of source code must retain the above copyright notice, this list of conditions and the following disclaimer.\n\n2. Redistributions in binary form must reproduce the above copyright notice, this list of conditions and the following disclaimer in the documentation and/or other materials provided with the distribution.\n\n3. Neither the name of the copyright holder nor the names of its contributors may be used to endorse or promote products derived from this software without specific prior written permission.\n\nTHIS SOFTWARE IS PROVIDED BY THE COPYRIGHT HOLDERS AND CONTRIBUTORS “AS IS” AND ANY EXPRESS OR IMPLIED WARRANTIES, INCLUDING, BUT NOT LIMITED TO, THE IMPLIED WARRANTIES OF MERCHANTABILITY AND FITNESS FOR A PARTICULAR PURPOSE ARE DISCLAIMED. IN NO EVENT SHALL THE COPYRIGHT HOLDER OR CONTRIBUTORS BE LIABLE FOR ANY DIRECT, INDIRECT, INCIDENTAL, SPECIAL, EXEMPLARY, OR CONSEQUENTIAL DAMAGES (INCLUDING, BUT NOT LIMITED TO, PROCUREMENT OF SUBSTITUTE GOODS OR SERVICES; LOSS OF USE, DATA, OR PROFITS; OR BUSINESS INTERRUPTION) HOWEVER CAUSED AND ON ANY THEORY OF LIABILITY, WHETHER IN CONTRACT, STRICT LIABILITY, OR TORT (INCLUDING NEGLIGENCE OR OTHERWISE) ARISING IN ANY WAY OUT OF THE USE OF THIS SOFTWARE, EVEN IF ADVISED OF THE POSSIBILITY OF SUCH DAMAGE."
  n1 = call "AlliGator Event to String.vi"("AlliGator Q Event"="AlliGator Q Event in") -> ("String"=w6:string)  [unwired: 8 in]
  n2 = case shown="\"Decay Fit Parameter Map:Change Decay Fit Parameter Map Color Palette\"" "AlliGator Q Event in" {
    selector: "AlliGator Q Event in" -> [_ _ w65 _ _ _ _ _ _ _ _ _ _ _ _]
    tunnel: "Data" -> [w29 w33 w66 _ w131 w163 w176 w189 w205 w228 w236 _ _ w267 w276]
    tunnel: "AlliGator Q Elements in" -> [w30 w49 w62 w118 w132 w165 w179 w194 w210 w229 w237 w242 w249 w270 w279]
    tunnel: [w30 w48 w62 w118 w132 w165 w179 w194 w210 w229 w237 w242 w248 w269 w278] -> w8
    tunnel: "VI in" -> [w18 w39 _ w115 w124 _ w171 w187 w203 _ _ _ w246 _ _]
    tunnel: "Script in" -> [w17 w50 w56 w110 w119 w134 w166 w180 w197 w217 w230 w238 w244 w271 w280]
    tunnel: w6 -> [w20 w31 _ w116 w128 _ w177 w192 w208 _ _ _ w243 _ _]
    tunnel: "error in (no error)" -> [w23 _ _ _ _ _ _ _ _ _ _ w241 _ w264 w274]
    tunnel: [w19 w42 w57 w117 w129 w135 w178 w193 w209 w218 w231 w241 w245 w268 w277] -> w13
    tunnel: "AlliGator Ctrl Refnums" -> [w25 w41 w61 _ w126 w150 _ w190 w206 w225 _ _ w247 _ _]
    tunnel: "data value reference" -> [w28 w37 w58 w113 w122 w140 w169 w182 w199 w220 w234 w240 w251 w272 w281]
    tunnel: [w27 w36 w58 w114 w123 w138 w170 w183 w200 w220 w233 w240 w250 w272 w281] -> w16
    tunnel: [w22 _ w55 _ _ w136 _ _ _ w219 _ _ _ _ _] -> w3
    tunnel: [w17 w50 w56 w110 w119 w134 w166 w180 w197 w217 w230 w238 w244 w271 w280] -> w5
    frame "Decay Fit Parameter Map:Export ROI NLSF Data as ASCII", Default {
      n3 = call-poly "Variant to Data.vi"("Variant"=w29) -> ("Value"=w26:bool)  [unwired: 8 in]
      n4 = call "Show Animated Busy Icon with Message.vi"("Already active? (F)"=w17, "Message"=w20, "Error In"=w23, "Target VI Refnum"=w18) -> ("Error Out"=w21:errorcluster)  [unwired: 7 in]
      n5 = call "AlliGator Export ROI(s) NLSF Parameters as ASCII File.vi"("AlliGator Ctrl Refnums"=w25, "error in (no error)"=w21, "All ROIs"=w26, "AlliGator IV DVR in"=w28) -> ("error out"=w24:errorcluster, "Message"=w22:string, "AlliGator IV DVR out"=w27:refnum<data-value>)  [unwired: 5 in]
      n6 = call "Hide Animated Busy Icon with Message.vi"("Already active? (F)"=w17, "Error In"=w24, "Target VI reference"=w18) -> ("Error Out"=w19:errorcluster)  [unwired: 8 in]
    }
    frame "Decay Fit Parameter Map:Build Decay Fit Parameter Map" {
      # "\"Build Decay Fit Parameter Map\""
      n7 = Unbundle By Name(w41) -> ("Decay Fit Map Ctrl Refums"=w38:T13)
      n8 = Variant To Data(Variant=w33) -> (data=w34:T21, error out=w32:errorcluster)  [unwired: 2 in]
      n9 = call "Show Animated Busy Icon with Message and Abort Button.vi"("Already active? (F)"=w50, "Message"=w31, "Target VI reference"=w39, "Error In"=w32) -> ("Error Out"=w40:errorcluster)  [unwired: 15 in]
      n10 = call "AlliGator Build Decay Fit Parameter Map.vi"("error in (no error)"=w40, "Decay Fit Parameter Map Update Event Data"=w34, "Decay Fit Map Ctrl Refums"=w38, "AlliGator Internal Variables DVR"=w37) -> ("error out"=w47:errorcluster, "AlliGator Internal Variables DVR"=w36:refnum<data-value>)  [unwired: 2 in, 4 out]
      n11 = call "Hide Animated Busy Icon with Message and Abort Button.vi"("Already active? (F)"=w50, "Target VI reference"=w39, "Error In"=w47) -> ("Error Out"=w35:errorcluster)  [unwired: 16 in]
      n12 = Bundle By Name(cluster=T4 {"AlliGator Q Event"=enum."Decay Fit Parameter Map:Change Decay Fit Parameter Map Color Palette", "Data"=variant} ("Alligator Atomic Action"), "Data"="Refresh Image") -> (w43:T4)
      n13 = call-poly "AlliGator Add Action(s) to Stack.vi"("Elements Order in Action Stack (Default: 2 BEFORE 1)"=Alligator_Elements_Order_in_Action_Stack."Enqueue 2 BEFORE 1", "Error In"=w35, "Alligator Atomic Action"=w43, "Alligator Queue Element 1"=w49) -> ("Error Out"=w42:errorcluster, "Alligator Queue Element 1 (+ 2)"=w48:T4[])  [unwired: 6 in]
    }
    frame "Decay Fit Parameter Map:Change Decay Fit Parameter Map Color Palette" {
      w51 = AlliGator_Variables_List."Decay Fit Parameter Map Palette List" ("Alligator Variable")
      # "\"Change Decay Fit Parameter Map Color Palette\""
      n14 = call "Alligator Variables Storage.vi"("Get(F)/Set"=FALSE, "AlliGator Variable"=w51) -> ("Data out"=w54:variant)  [unwired: 7 in, 2 out]
      n15 = call-poly "Variant to Data.vi"("Variant"=w54) -> ("String Array"=w52:string[])  [unwired: 8 in]
      n16 = call-poly "Variant to Data.vi"("Variant"=w66) -> ("String"=w64:string)  [unwired: 8 in]
      n17 = Unbundle By Name(w61) -> ("Decay Fit Map Ctrl Refums"=w60:T13)
      n18 = case shown="\"Edit Palette List...\"" w64 {
        selector: w64 -> [_ w93 _]
        tunnel: w65 -> [_ _ _]
        tunnel: [w72 w77 w106] -> w63
        tunnel: [w71 w85 w104] -> w59
        tunnel: ["Palette List Edited" ("Append to Message") w84 _] -> w55
        tunnel: w52 -> [w68 w81 _]
        tunnel: w51 -> [w67 w76 _]
        frame "Edit Palette List..." {
          n19 = call "Edit Image Palette List Dialog.vi"("Palette List (in)"=w68) -> ("Palette List (out)"=w75:string[])  [unwired: 10 in]
          n20 = call "Alligator Variables Storage.vi"("Get(F)/Set"=TRUE, "AlliGator Variable"=w67, "Data in"=w75) -> ("Error Out"=w73:errorcluster)  [unwired: 6 in, 2 out]
          n21 = call "AlliGator Check Selected Palette.vi"("Error In"=w73, "Image"=AlliGator_Image_Display_Type."Decay Fit Parameter Map") -> ("Error Out"=w72:errorcluster, "Image Display Palette Information"=w71:T17)  [unwired: 8 in]
        }
        frame Default {
          n22 = call "Get User Palette Choice.vi"("Palette"=w93) -> ("Error Out"=w89:errorcluster, "Palette Colors"=w91:u32[], "Palette Type"=w92:T18, "Palette Name (# Colors)"=w79:string, "Interpolate?"=w87:bool, "Built-in Palette?"=w80:bool)  [unwired: 3 in, 2 out]
          n23 = Format Into String(format string="%s", initial string="Palette selected: ", w79) -> (resulting string=w84:string)  [unwired: 1 in, 1 out]
          n24 = Bundle(cluster=T17 {"Palette Name [# Colors,int?,inv?]"="", "Palette Type"=0, "Palette Colors"=[], "Interpolate?"=FALSE} ("Image Display Palette Information"), "Palette Name [# Colors,int?,inv?]"=w79, "Palette Type"=w92, "Palette Colors"=w91, "Interpolate?"=w87) -> (w85:T17)
          n25 = call "Alligator Variables Storage.vi"("Get(F)/Set"=TRUE, "AlliGator Variable"=AlliGator_Variables_List."Decay Fit Parameter Map Palette Information" ("Alligator Variable"), "Error In"=w89, "Data in"=w85) -> ("Error Out"=w78:errorcluster)  [unwired: 5 in, 2 out]
          n26 = case shown="False" w80 {
            tunnel: w78 -> [w101 w102]
            tunnel: [w100 w102] -> w77
            tunnel: w79 -> [w99 _]
            tunnel: w81 -> [w98 _]
            tunnel: w76 -> [w96 _]
            frame False {
              n27 = Build Array (concatenate)(w98, w99) -> (w97:string[])
              n28 = call "Remove Duplicates From 1D Array.vim"("array"=w97) -> ("array with duplicates removed"=w95:string[])  [unwired: 10 in]
              n29 = call "Alligator Variables Storage.vi"("Get(F)/Set"=TRUE, "AlliGator Variable"=w96, "Error In"=w101, "Data in"=w95) -> ("Error Out"=w100:errorcluster)  [unwired: 5 in, 2 out]
            }
            frame True {
            }
          }
        }
        frame "Refresh Image" {
          n30 = call "Alligator Variables Storage.vi"("Get(F)/Set"=FALSE, "AlliGator Variable"=AlliGator_Variables_List."Decay Fit Parameter Map Palette Information" ("Alligator Variable")) -> ("Error Out"=w107:errorcluster, "Data out"=w108:variant)  [unwired: 7 in, 1 out]
          n31 = Variant To Data(error in=w107, type=T17 {"Palette Name [# Colors,int?,inv?]"="", "Palette Type"=0, "Palette Colors"=[], "Interpolate?"=FALSE} ("Image Display Palette Information"), Variant=w108) -> (data=w104:T17, error out=w106:errorcluster)
        }
      }
      n32 = call "AlliGator Update Decay Fit Parameter Map Palette.vi"("error in (no error)"=w63, "Image Display Palette Information"=w59, "Decay Fit Map Ctrl Refums"=w60) -> ("error out"=w57:errorcluster)  [unwired: 8 in]
    }
    frame "Decay Fit Parameter Map:Export All Decay Fit Parameter Maps Data as ASCII" {
      # "\"Export All Decay Fit Parameter Maps Data as ASCII\""
      n33 = call "Show Animated Busy Icon with Message.vi"("Already active? (F)"=w110, "Message"=w116, "Target VI Refnum"=w115) -> ("Error Out"=w111:errorcluster)  [unwired: 8 in]
      n34 = call "AlliGator Save All Decay Fit Parameter Maps to ASCII.vi"("error in (no error)"=w111, "Data Value Reference in"=w113) -> ("error out"=w112:errorcluster, "Data Value Reference out"=w114:refnum<data-value>)  [unwired: 8 in]
      n35 = call "Hide Animated Busy Icon with Message.vi"("Already active? (F)"=w110, "Error In"=w112, "Target VI reference"=w115) -> ("Error Out"=w117:errorcluster)  [unwired: 8 in]
    }
    frame "Decay Fit Parameter Map:Export Decay Fit Parameter Map Data as ASCII" {
      # "\"Export Decay Fit Parameter Map Data as ASCII\""
      n36 = call-poly "Variant to Data.vi"("Variant"=w131) -> ("Value"=w130:bool)  [unwired: 8 in]
      n37 = Unbundle By Name(w126) -> ("Decay Fit Map Ctrl Refums.Decay Fit Parameter"=w127:refnum<vi>)
      n38 = property class="Enum (strict)"(reference=w127) -> ("Value"=w125:T20)  [unwired: 1 in, 2 out]
      n39 = call "Show Animated Busy Icon with Message.vi"("Already active? (F)"=w119, "Message"=w128, "Target VI Refnum"=w124) -> ("Error Out"=w121:errorcluster)  [unwired: 8 in]
      n40 = call "AlliGator Save Decay Fit Parameter Map to ASCII.vi"("Fit Parameter"=w125, "error in (no error)"=w121, "Dialog?"=w130, "Data Value Reference in"=w122) -> ("error out"=w120:errorcluster, "Data Value Reference out"=w123:refnum<data-value>)  [unwired: 6 in]
      n41 = call "Hide Animated Busy Icon with Message.vi"("Already active? (F)"=w119, "Error In"=w120, "Target VI reference"=w124) -> ("Error Out"=w129:errorcluster)  [unwired: 8 in]
    }
    frame "Decay Fit Parameter Map:Save Decay Fit Parameter Map Image" {
      # "\"Save Decay Fit Parameter Map Image\""
      n42 = Unbundle By Name(w150) -> ("Registered Events Ctrl Refnums.Decay Fit Parameter Map Display"=w164:refnum<vi>, "Decay Fit Map Ctrl Refums.Decay Fit Parameter"=w149:refnum<vi>)
      n43 = call-poly "Variant to Data.vi"("Variant"=w163) -> ("Value"=w157:bool)  [unwired: 8 in]
      n44 = call "AlliGator IV Dataset Path.vi"("Get (F)/ Set (T)"=FALSE, "AlliGator IV DVR in"=w140) -> ("error out"=w137:errorcluster, "[Time-Series Path]"=w142:path[], "Single Data Point Path"=w143:path, "AlliGator IV DVR out"=w138:refnum<data-value>, "Current Dataset"=w141:i32)  [unwired: 5 in]
      n45 = call "AlliGator Get Image File Format.vi"("Error In"=w137) -> ("error out"=w154:errorcluster, "Transparent Mask Color"=w133:u32, "File Extension (.xxx)"=w151:string, "Image File Format"=w159:T22)  [unwired: 7 in]
      n46 = call "AlliGator Get Destination Folder.vi"("Current Data Set (-1: single)"=w141, "Time-Series Paths"=w142, "Single Data Point Path"=w143) -> ("Data Point Name"=w156:string, "Destination Folder path"=w162:path)  [unwired: 6 in, 1 out]
      n47 = property class="Enum (strict)"(reference=w149) -> ("Value"=w148:T20)  [unwired: 1 in, 2 out]
      n48 = Format Into String(format string=" %s Map%s", initial string=w156, error in=w154, w148, w151) -> (resulting string=w153:string, error out=w152:errorcluster)
      n49 = Build Path(base path=w162, name or relative path=w153) -> (appended path=w161:path)
      n50 = call "Image File Dialog (Optional).vi"("Dialog?"=w157, "Error In"=w152, "Image File Format in"=w159, "Default file path in"=w161) -> ("Error Out"=w144:errorcluster, "Image File Format out"=w158:T22, "file path out"=w160:path)  [unwired: 5 in]
      n51 = call "Image Display Save Image.vi"("Mask Color (Transparent)"=w133, "error in (no error)"=w144, "Saved Image File Format"=w158, "File Path in"=w160, "Display Image Control Refnum"=w164) -> ("Error Out"=w145:errorcluster, "File Path out"=w146:path)  [unwired: 5 in]
      n52 = Format Into String(format string="Decay Fit Parameter Map Image saved to %s", error in=w145, w146) -> (resulting string=w136:string, error out=w135:errorcluster)  [unwired: 1 in]
    }
    frame "Decay Fit Parameter Map:Save-Load IRFs & Fit Data" {
      # "\"Save-Load IRFs & Fit Data\""
      n53 = Variant To Data(type=T19 {"Load/Save"=FALSE, "File Path"=path ""} ("Calibration File Information"), Variant=w176) -> (data=w174:T19)  [unwired: 1 in, 1 out]
      n54 = Unbundle By Name(w174) -> ("File Path"=w173:path, "Load/Save"=w172:bool)
      n55 = call "Show Animated Busy Icon with Message.vi"("Already active? (F)"=w166, "Message"=w177, "Target VI Refnum"=w171) -> ("Error Out"=w168:errorcluster)  [unwired: 8 in]
      n56 = call "AlliGator Save-Load IRFs & Fit Data (Map).vi"("error in (no error)"=w168, "Write(T)/Load (F)"=w172, "File Path"=w173, "Data Value Reference in"=w169) -> ("error out"=w167:errorcluster, "Data Value Reference out"=w170:refnum<data-value>)  [unwired: 6 in]
      n57 = call "Hide Animated Busy Icon with Message.vi"("Already active? (F)"=w166, "Error In"=w167, "Target VI reference"=w171) -> ("Error Out"=w178:errorcluster)  [unwired: 8 in]
    }
    frame "Decay Fit Parameter Map:Send Map Data to Lifetime Graph" {
      # "Send Map Data to Lifetime Graph"
      n58 = call-poly "Variant to Data.vi"("Variant"=w189) -> ("Value"=w188:i32)  [unwired: 8 in]
      n59 = Unbundle By Name(w190) -> ("Registered Events Ctrl Refnums.Lifetime Graph"=w191:refnum<vi>, "Decay Fit Map Ctrl Refums.Decay Fit Parameter"=w186:refnum<vi>)
      n60 = property class="Enum (strict)"(reference=w186) -> ("Value"=w185:T20)  [unwired: 1 in, 2 out]
      n61 = call "Show Animated Busy Icon with Message.vi"("Already active? (F)"=w180, "Message"=w192, "Target VI Refnum"=w187) -> ("Error Out"=w184:errorcluster)  [unwired: 8 in]
      n62 = call "AlliGator Send Decay Fit Parameter Map to Lifetime Graph.vi"("Fit Parameter"=w185, "Lifetime Graph refnum"=w191, "error in (no error)"=w184, "ROI idx (2147483647: all ROIs)"=w188, "Data Value Reference in"=w182) -> ("error out"=w181:errorcluster, "Data Value Reference out"=w183:refnum<data-value>)  [unwired: 5 in]
      n63 = call "Hide Animated Busy Icon with Message.vi"("Already active? (F)"=w180, "Error In"=w181, "Target VI reference"=w187) -> ("Error Out"=w193:errorcluster)  [unwired: 8 in]
    }
    frame "Decay Fit Parameter Map:Plot Map Data vs Intensity" {
      # "\"Decay Fit Parameter Map:Plot Map Data vs Intensity\""
      n64 = call-poly "Variant to Data.vi"("Variant"=w205) -> ("Value"=w204:i32)  [unwired: 8 in]
      n65 = Unbundle By Name(w206) -> ("Registered Events Ctrl Refnums.Lifetime Graph"=w207:refnum<vi>, "Decay Fit Map Ctrl Refums.Decay Fit Parameter"=w202:refnum<vi>)
      n66 = property class="Enum (strict)"(reference=w202) -> ("Value"=w201:T20)  [unwired: 1 in, 2 out]
      n67 = call "Show Animated Busy Icon with Message.vi"("Already active? (F)"=w197, "Message"=w208, "Target VI Refnum"=w203) -> ("Error Out"=w196:errorcluster)  [unwired: 8 in]
      n68 = disable-structure shown="Disabled" {
        disable-tunnel: w196 -> [w215 w216]
        disable-tunnel: [w214 w216] -> w195
        frame Disabled {
          n69 = call "Two Button Dialog with Error.vi"("Error In"=w215, "F button name (\"Cancel\")"="No" ("F button name (\"Cancel\")"), "T button name (\"OK\")"="Yes" ("T button name (\"OK\")"), "message"="Use baseline-subtracted intensity?") -> ("Error Out"=w214:errorcluster)  [unwired: 6 in, 1 out]
        }
        frame Enabled {
        }
      }
      n70 = call "AlliGator Plot Fit Parameter vs Intensity v2.vi"("Fit Parameter"=w201, "Lifetime Graph refnum"=w207, "error in (no error)"=w195, "ROI idx (2147483647: all ROIs)"=w204, "Data Value Reference in"=w199) -> ("error out"=w198:errorcluster, "Data Value Reference out"=w200:refnum<data-value>)  [unwired: 5 in]
      n71 = call "Hide Animated Busy Icon with Message.vi"("Already active? (F)"=w197, "Error In"=w198, "Target VI reference"=w203) -> ("Error Out"=w209:errorcluster)  [unwired: 8 in]
    }
    frame "Decay Fit Parameter Map:Set Decay Fit  Parameter Map Selection" {
      # "used in script"
      # "\"Decay Fit  Parameter Map:Set Decay Fit  Parameter Map Selection\""
      n72 = Unbundle By Name(w225) -> ("Decay Fit Map Ctrl Refums.Decay Fit Parameter"=w224:refnum<vi>)
      n73 = Variant To Data(type=Decay_Fit_Parameters_&_Derived_Quantities_List."Offset" ("Fit Parameter"), Variant=w228) -> (data=w223:T20, error out=w222:errorcluster)  [unwired: 1 in]
      n74 = property class="Enum (strict)"(reference=w224, error in=w222, "Value"=w223) -> (error out=w221:errorcluster)  [unwired: 1 out]
      n75 = Format Into String(format string="Decay Fit Parameter Map Selection set to %s", error in=w221, w223) -> (resulting string=w219:string, error out=w218:errorcluster)  [unwired: 1 in]
    }
    frame "Decay Fit Parameter Map:Update Local Decay Plots" {
      # "\"Update Local Decay Plots\""
      n76 = Variant To Data(Variant=w236) -> (data=w235:T23, error out=w232:errorcluster)  [unwired: 2 in]
      n77 = call "AlliGator Send Local Decay Plots.vi"("error in (no error)"=w232, "ROI Descriptor"=w235, "AlliGator IV DVR in"=w234) -> ("error out"=w231:errorcluster, "AlliGator IV DVR out"=w233:refnum<data-value>)  [unwired: 7 in]
    }
    frame "Decay Fit Parameter Map:Python Function Decay Fit Parameters Map Event" {
      # "\"Decay Fit Parameters:Python Function Decay Fit Parameters Map Event\""
      n78 = One Button Dialog(message="Not yet supported....") -> ()  [unwired: 1 in, 1 out]
      n79 = call "Play Error Sound.vi"() -> ()  [unwired: 27 in, 1 out]
    }
    frame "Decay Fit Parameter Map:Overlay Decay Fit Parameter Map in Source Image" {
      # "\"Overlay Decay Fit Parameter Map in Source Image\""
      n80 = Unbundle By Name(w247) -> ("Decay Fit Map Ctrl Refums.Decay Fit Parameter Map Color Scale"=w257:refnum<vi>, "Dataset Control References.Image Color Scale"=w258:refnum<vi>, "Registered Events Ctrl Refnums.Source Image Display"=w256:refnum<vi>)
      n81 = Unbundle By Name(w247) -> ("Dataset Control References.Save Image"=w255:refnum<vi>)
      n82 = call "Show Animated Busy Icon with Message.vi"("Already active? (F)"=w244, "Message"=w243, "Target VI Refnum"=w246) -> ("Error Out"=w253:errorcluster)  [unwired: 8 in]
      n83 = property class="Bool (strict)"(reference=w255) -> ("Value"=w254:bool)  [unwired: 1 in, 2 out]
      n84 = case shown="True" w254 {
        tunnel: w249 -> [w259 w263]
        tunnel: [w259 w260] -> w248
        frame False {
        }
        frame True {
          n85 = call-poly "AlliGator Add Action(s) to Stack.vi"("Elements Order in Action Stack (Default: 2 BEFORE 1)"=Alligator_Elements_Order_in_Action_Stack."Enqueue 2 BEFORE 1", "Alligator Atomic Action"=T4 {"AlliGator Q Event"=enum."Image:Save Displayed Image with Overlay", "Data"=variant}, "Alligator Queue Element 1"=w263) -> ("Alligator Queue Element 1 (+ 2)"=w260:T4[])  [unwired: 7 in, 1 out]
        }
      }
      n86 = call "AlliGator Color Decay Fit Parameter Map in Original Image.vi"("Decay Fit Parameter Map Color Scale Refnum"=w257, "Image Color Scale Refnum"=w258, "Error In"=w253, "Destination Image Control Refnum"=w256, "AlliGator IV DVR in"=w251) -> ("Error Out"=w252:errorcluster, "AlliGator IV DVR out"=w250:refnum<data-value>)  [unwired: 4 in, 1 out]
      n87 = call "Hide Animated Busy Icon with Message.vi"("Already active? (F)"=w244, "Error In"=w252, "Target VI reference"=w246) -> ("Error Out"=w245:errorcluster)  [unwired: 8 in]
    }
    frame "Decay Fit Parameter Map:Mouse Up" {
      # "\"Decay Fit Parameter Map:Mouse Up\""
      n88 = Variant To Data(error in=w264, Variant=w267) -> (data=w266:T24, error out=w265:errorcluster)  [unwired: 1 in]
      n89 = call "AlliGator Decay Parameters Map Mouse Up Event.vi"("error in (no error)"=w265, "Image Control Refnum"=w266, "AlliGator Actions in"=w270) -> ("error out"=w268:errorcluster, "AlliGator Actions out"=w269:T4[])  [unwired: 7 in]
    }
    frame "Decay Fit Parameter Map:Display Range Mouse Move" {
      # "\"Decay Fit Parameter Map:Display Range Mouse Move\""
      n90 = Variant To Data(error in=w274, Variant=w276) -> (data=w275:T20, error out=w273:errorcluster)  [unwired: 1 in]
      n91 = call "AlliGator Decay Parameter Range Mouse Move Event.vi"("Error In"=w273, "Decay Fit Parameter"=w275, "AlliGator Actions in"=w279) -> ("Error Out"=w277:errorcluster, "AlliGator Actions out"=w278:T4[])  [unwired: 7 in]
    }
  }
  "Data Value Reference out" <- w16
  "error out" <- w13
  "AlliGator Q Elements out" <- w8
  "Script out" <- w5
  n92 = call "Message Style.vi"() -> ("Message Formatting"=w2:T2)
  n93 = call "AlliGator Package Notebook Messages.vi"("Message Formatting"=w2, "Message"=w3, "AlliGator Q Event in"="AlliGator Q Event in") -> ("[Notebook Message]"=→"[Notebook Message]":T1[])  [unwired: 8 in]
